vi "Get Process Lookup.vi"(8 "error in (no error)":errorcluster, 11 "CD_Process in":refnum<class "CD_Process.lvclass">) -> (0 "error out":errorcluster, 3 "CD_Process out":refnum<class "CD_Process.lvclass">)   [LabVIEW 2019, in "TimingDRV Engine.lvlib" / "CD_Process.lvclass"]
uses:
  CD_Process.lvclass
  TypeDefs/Process Lookup.ctl
  TypeDefs/Message.ctl
  CD_Process.lvclass/CD_Process.ctl
panel:
  out "Process Lookup":T1
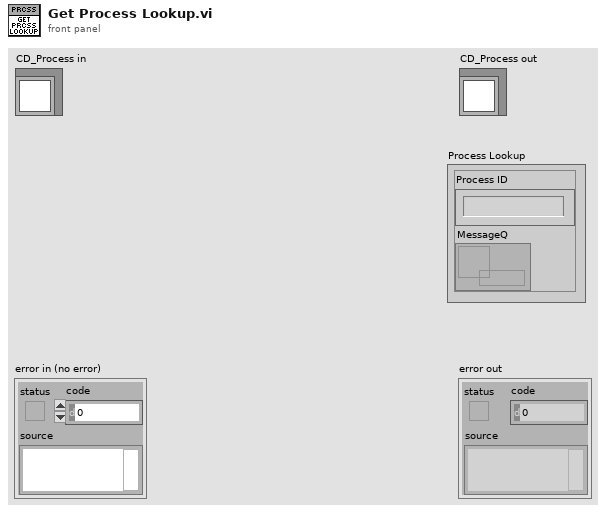
[diagram p1: front panel]
types:
  T1 = typedef "TimingDRV Engine.lvlib/CD_Process.lvclass/Process Lookup.ctl" = cluster{"Process ID":string, "MessageQ":refnum<queue>}
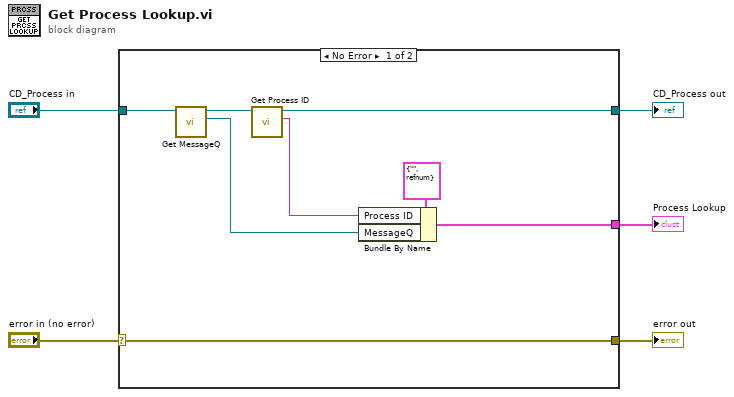
[diagram p0: block diagram]
diagram:
  n1 = case shown="No Error" "error in (no error)" {
    selector: "error in (no error)" -> [w13 w15]
    tunnel: [w13 w15] -> w4
    tunnel: [w7 w14] -> w2
    tunnel: "CD_Process in" -> [w8 w14]
    tunnel: [w6 _] -> w1
    frame No Error {
      n2 = call "Get MessageQ.vi"("CD_Process in"=w8) -> ("MessageQ"=w9:refnum<queue>, "CD_Process out"=w11:refnum<class "CD_Process.lvclass">)  [unwired: 9 in]
      n3 = call "Get Process ID.vi"("CD_Process in"=w11) -> ("Process ID"=w10:string, "CD_Process out"=w7:refnum<class "CD_Process.lvclass">)  [unwired: 9 in]
      n4 = Bundle By Name(cluster=T1 {"Process ID"="", "MessageQ"=refnum} ("Process Lookup"), "Process ID"=w10, "MessageQ"=w9) -> (w6:T1)
    }
    frame Error {
    }
  }
  "error out" <- w4
  "CD_Process out" <- w2
  "Process Lookup" <- w1
